vi "fnInfoRange.vi"(1 "eEng2":dbl[](array[numeric]), 2 "dData2":dbl[](array[numeric]), 3 "eEng1":dbl[](array[numeric]), 4 "dData1":dbl[](array[numeric])) -> (0 "返回类型":i32)   [LabVIEW 2012]
uses:
  LabView4Las.dll
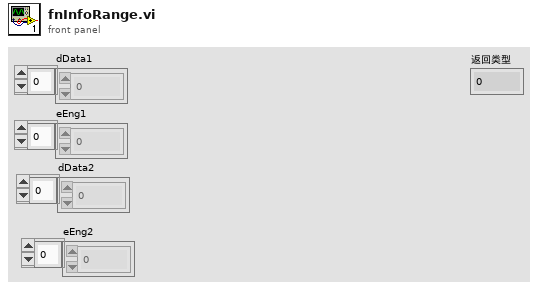
[diagram p1: front panel]
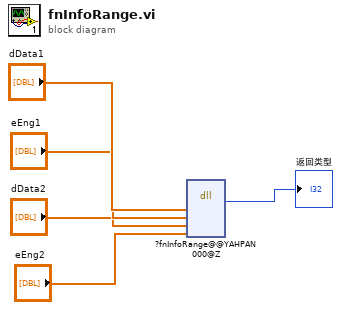
[diagram p0: block diagram]
diagram:
  n1 = dll-call lib="C:/Developer/labview/dll2/LabView4Las.dll" fn="?fnInfoRange@@YAHPAN000@Z"("dData1"="dData1", "eEng1"="eEng1", "dData2"="dData2", "eEng2"="eEng2") -> ("返回类型"=→"返回类型":i32)  [unwired: 7 in, 2 out]
